vi "Read Video Frame.vi"(8 "error in (no error)":errorcluster, 11 "Frame Data Message in":refnum<class "Frame Data Message.lvclass">) -> (0 "error out":errorcluster, 2 "Video Frame.lvclass":refnum<class "Video Frame.lvclass">, 3 "Frame Data Message out":refnum<class "Frame Data Message.lvclass">)   [LabVIEW 2018, in "Frame Data Message.lvclass"]
uses:
  Frame Data Message.lvclass
  Video Frame/Video Frame.lvclass
  Frame Data Message.lvclass/Frame Data Message.ctl
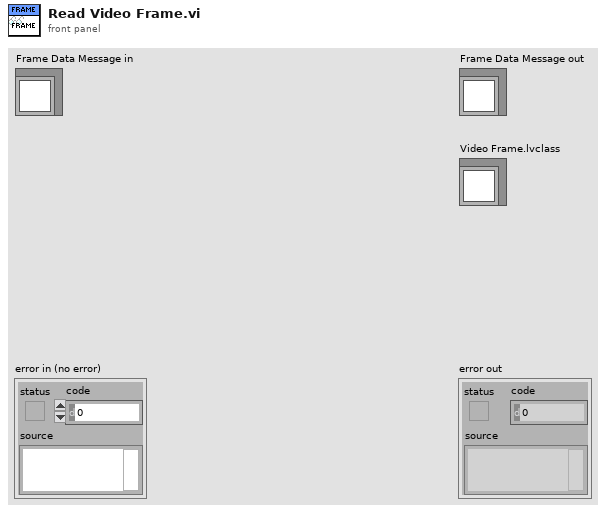
[diagram p1: front panel]
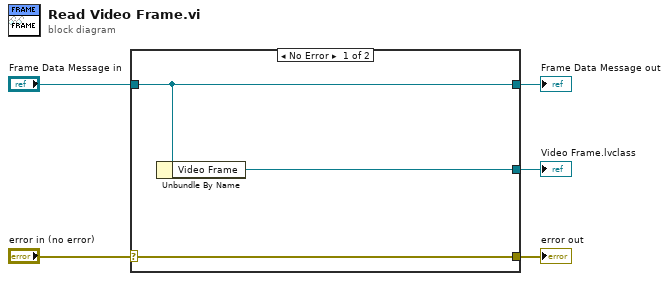
[diagram p0: block diagram]
diagram:
  n1 = case shown="No Error" "error in (no error)" {
    selector: "error in (no error)" -> [w8 w9]
    tunnel: [w8 w9] -> w4
    tunnel: [w7 w10] -> w2
    tunnel: "Frame Data Message in" -> [w7 w10]
    tunnel: [w6 _] -> w1
    frame No Error {
      n2 = Unbundle By Name(w7) -> ("Video Frame"=w6:refnum<class "Video Frame.lvclass">)
    }
    frame Error {
    }
  }
  "error out" <- w4
  "Frame Data Message out" <- w2
  "Video Frame.lvclass" <- w1
